vi "FindMassResolution_Multiple.vi"(7 "EnableResDisplay":bool, 10 "BinnedSpectrum":cluster{"m/z Array":dbl[], "Signal":dbl[]}, 11 "GraphRef.":refnum<vi>) -> (2 "FWHM":dbl, 3 "Resolution":dbl)   [LabVIEW 2012]
uses:
  <vilib>/Utility/miscctls.llb/LVCursorListTypeDef.ctl
  <vilib>/Utility/miscctls.llb/LVAnnotationListTypeDef.ctl
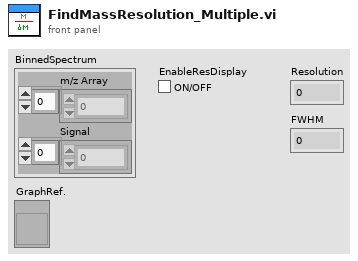
[diagram p1: front panel]
types:
  T1 = typedef "LVAnnotationListTypeDef.ctl" = cluster{"Name":string, "Color":u32, "Style":u8, "Point Style":u8, "Name Visible":bool, "Allow Drag":bool, "Annotation Mode":u32, "Plot":i32, "Index":i32, "Position":cluster{"X":dbl, "Y":dbl}, "X Scale":u32, "Y Scale":u32, "Show Arrow":bool, "Lock Name":bool, "Plot Area":i32, "Label Offset":cluster{"X":dbl, "Y":dbl}}[]
  T2 = typedef "LVCursorListTypeDef.ctl" = cluster{"Name":string, "Color":u32, "Style":u8, "Point Style":u8, "Name Visible":bool, "Allow Drag":bool, "Cursor Mode":u32, "Plot":i32, "Index":i32, "Position":cluster{"X":dbl, "Y":dbl}, "X Scale":u32, "Y Scale":u32, "Watch Plots":i32[], "Watch All Plots":bool, "Plot Area":i32, "Label Offset":cluster{"X":dbl, "Y":dbl}}[]
  T3 = cluster{"Name":string, "Color":u32, "Style":u8, "Point Style":u8, "Name Visible":bool, "Allow Drag":bool, "Annotation Mode":u32, "Plot":i32, "Index":i32, "Position":cluster{"X":dbl, "Y":dbl}, "X Scale":u32, "Y Scale":u32, "Show Arrow":bool, "Lock Name":bool, "Plot Area":i32, "Label Offset":cluster{"X":dbl, "Y":dbl}}
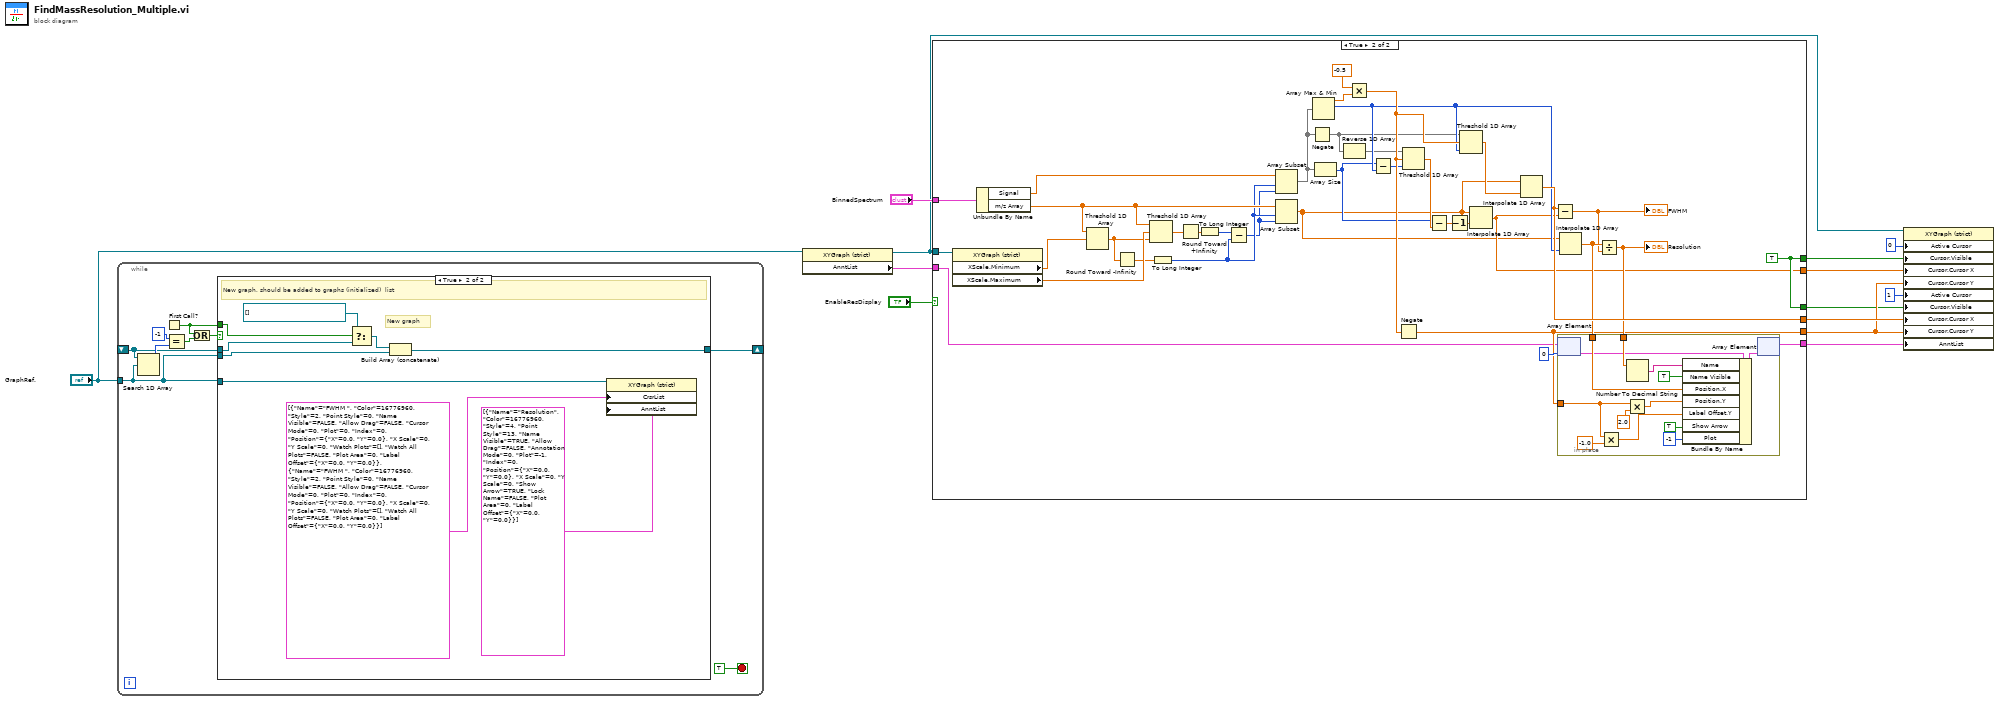
[diagram p0: block diagram]
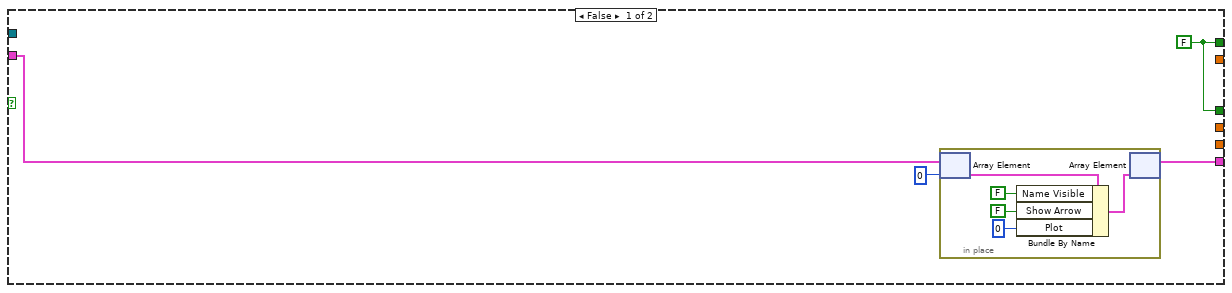
[diagram p2: hidden frame]
diagram:
  n1 = while {
    tunnel: "GraphRef." -> [w19]
    shift-right: [w18] -> _
    shift-left: _ -> [w17]
    stop <- TRUE stop-if-true
    n2 = Search 1D Array(1D array=w17, element=w19) -> (index of element=w21:i32)  [unwired: 1 in]
    n3 = First Call?() -> (First Call?: T/F=w14:bool)
    n4 = Equal?(x=-1, y=w21) -> (x = y?=w20:bool)
    n5 = Or(x=w14, y=w20) -> (x .or. y?=w15:bool)
    n6 = case shown="True" w15 {
      tunnel: w17 -> [w23 w28]
      tunnel: [w23 w32] -> w18
      tunnel: w19 -> [_ w31]
      tunnel: w19 -> [_ w30]
      tunnel: w14 -> [_ w25]
      frame False {
      }
      frame True {
        # "New graph"
        # "New graph, should be added to graphs (initialized)  list"
        n7 = Select(t=refnum<vi>[] [], s=w25, f=w28) -> (s? t:f=w27:refnum<vi>[])
        n8 = Build Array (concatenate)(w27, w31) -> (w32:refnum<vi>[])
        n9 = property class="XYGraph (strict)"(reference=w30, "CrsrList"=T2 [{"Name"="FWHM ", "Color"=16776960, "Style"=2, "Point Style"=0, "Name Visible"=FALSE, "Allow Drag"=FALSE, "Cursor Mode"=0, "Plot"=0, "Index"=0, "Position"={"X"=0.0, "Y"=0.0}, "X Scale"=0, "Y Scale"=0, "Watch Plots"=[], "Watch All Plots"=FALSE, "Plot Area"=0, "Label Offset"={"X"=0.0, "Y"=0.0}}, {"Name"="FWHM ", "Color"=16776960, "Style"=2, "Point Style"=0, "Name Visible"=FALSE, "Allow Drag"=FALSE, "Cursor Mode"=0, "Plot"=0, "Index"=0, "Position"={"X"=0.0, "Y"=0.0}, "X Scale"=0, "Y Scale"=0, "Watch Plots"=[], "Watch All Plots"=FALSE, "Plot Area"=0, "Label Offset"={"X"=0.0, "Y"=0.0}}] ("Cursor List"), "AnntList"=T1 [{"Name"="Resolution", "Color"=16776960, "Style"=4, "Point Style"=13, "Name Visible"=TRUE, "Allow Drag"=FALSE, "Annotation Mode"=0, "Plot"=-1, "Index"=0, "Position"={"X"=0.0, "Y"=0.0}, "X Scale"=0, "Y Scale"=0, "Show Arrow"=TRUE, "Lock Name"=FALSE, "Plot Area"=0, "Label Offset"={"X"=0.0, "Y"=0.0}}] ("Annotation List")) -> ()  [unwired: 1 in, 2 out]
      }
    }
  }
  n10 = property class="XYGraph (strict)"(reference="GraphRef.") -> (reference out=w2:refnum<vi>, "AnntList"=w3:T1)  [unwired: 1 in, 1 out]
  n11 = case shown="True" "EnableResDisplay" {
    tunnel: "BinnedSpectrum" -> [_ w78]
    tunnel: w2 -> [_ w77]
    tunnel: [_ w49] -> w11
    tunnel: [_ w67] -> w10
    tunnel: [_ w50] -> w9
    tunnel: [w34 w55] -> w1
    tunnel: [w36 w54] -> w8
    tunnel: [w36 w54] -> w7
    tunnel: w3 -> [w33 w43]
    frame False {
      w36 = FALSE
      n12 = in-place {
        n13 = in-place-array #1(w33, 0) -> (w39:T3)
        n14 = Bundle By Name(cluster=w39, "Name Visible"=FALSE, "Show Arrow"=FALSE, "Plot"=0) -> (w41:T3)
        n15 = in-place-array #1(w41) -> (w34:T1)  [unwired: 1 out]
      }
    }
    frame True {
      w54 = TRUE
      n16 = property class="XYGraph (strict)"(reference=w77) -> ("XScale.Minimum"=w76:dbl, "XScale.Maximum"=w75:dbl)  [unwired: 1 in, 2 out]
      n17 = Unbundle By Name(w78) -> ("Signal"=w66:dbl[], "m/z Array"=w62:dbl[])
      n18 = Threshold 1D Array(2:w76, 3:w62) -> (0:w70:dbl)  [unwired: 1 in]
      n19 = Round Toward -Infinity(1:w70) -> (0:w72:dbl)
      n20 = Threshold 1D Array(1:w70, 2:w75, 3:w62) -> (0:w74:dbl)
      n21 = To Long Integer(number=w72) -> (32bit integer=w61:i32)
      n22 = Round Toward +Infinity(x=w74) -> (ceil(x): smallest int >= x=w73:dbl)
      n23 = To Long Integer(number=w73) -> (32bit integer=w71:i32)
      n24 = Subtract(x=w71, y=w61) -> (x-y=w60:i32)
      n25 = Array Subset(array=w66, index=w61, length=w60) -> (w53:dbl[])
      n26 = Array Subset(array=w62, index=w61, length=w60) -> (w46:dbl[])
      n27 = Negate(x=w53) -> (-x=w44:dbl[])
      n28 = Array Max & Min(array=w53) -> (max value=w69:dbl, max index (indices)=w51:i32)  [unwired: 2 out]
      n29 = Array Size(array=w53) -> (size(s)=w47:i32)
      n30 = Reverse 1D Array(array=w44) -> (reversed array=w45:dbl[])
      n31 = Multiply(x=-0.5, y=w69) -> (x*y=w57:dbl)
      n32 = Subtract(x=w47, y=w51) -> (x-y=w52:i32)
      n33 = Negate(x=w57) -> (-x=w50:dbl)
      n34 = Threshold 1D Array(1:w52, 2:w57, 3:w45) -> (0:w58:dbl)
      n35 = Subtract(x=w47, y=w58) -> (x-y=w48:dbl)
      n36 = Decrement(x=w48) -> (x-1=w42:dbl)
      n37 = Threshold 1D Array(1:w51, 2:w57, 3:w44) -> (0:w59:dbl)
      n38 = Interpolate 1D Array(1:w42, 2:w46) -> (0:w49:dbl)
      n39 = Interpolate 1D Array(1:w59, 2:w46) -> (0:w67:dbl)
      n40 = Subtract(x=w67, y=w49) -> (x-y=w63:dbl)
      "FWHM" <- w63
      n41 = Interpolate 1D Array(1:w51, 2:w46) -> (0:w65:dbl)
      n42 = Divide(x=w65, y=w63) -> (x/y=w56:dbl)
      "Resolution" <- w56
      n43 = in-place {
        in-place-border: w65 -> [w89]
        in-place-border: w50 -> [w83]
        in-place-border: w56 -> [w87]
        n44 = in-place-array #2(w43, 0) -> (w81:T3)
        n45 = Multiply(x=w83, y=-1.0) -> (x*y=w86:dbl)
        n46 = Number To Decimal String(number=w87) -> (decimal integer string=w88:string)  [unwired: 1 in]
        n47 = Multiply(x=w83, y=2.0) -> (x*y=w82:dbl)
        n48 = Bundle By Name(cluster=w81, "Name"=w88, "Name Visible"=TRUE, "Position.X"=w89, "Position.Y"=w82, "Label Offset.Y"=w86, "Show Arrow"=TRUE, "Plot"=-1) -> (w91:T3)
        n49 = in-place-array #2(w91) -> (w55:T1)  [unwired: 1 out]
      }
    }
  }
  n50 = property class="XYGraph (strict)"(reference=w2, "Active Cursor"=u32 0, "Cursor.Visible"=w8, "Cursor.Cursor X"=w11, "Cursor.Cursor Y"=w9, "Active Cursor"=u32 1, "Cursor.Visible"=w7, "Cursor.Cursor X"=w10, "Cursor.Cursor Y"=w9, "AnntList"=w1) -> ()  [unwired: 1 in, 2 out]
